vi "Write Subscribe Target.vi"(8 "error in (no error)":errorcluster, 10 "Subscribe Target":string, 11 "Subscriber in":refnum<class "Subscriber.lvclass">) -> (0 "error out":errorcluster, 3 "Subscriber out":refnum<class "Subscriber.lvclass">)   [LabVIEW 2024, in "Subscriber.lvclass"]
uses:
  Subscriber.lvclass
  Subscriber.lvclass/Subscriber.ctl
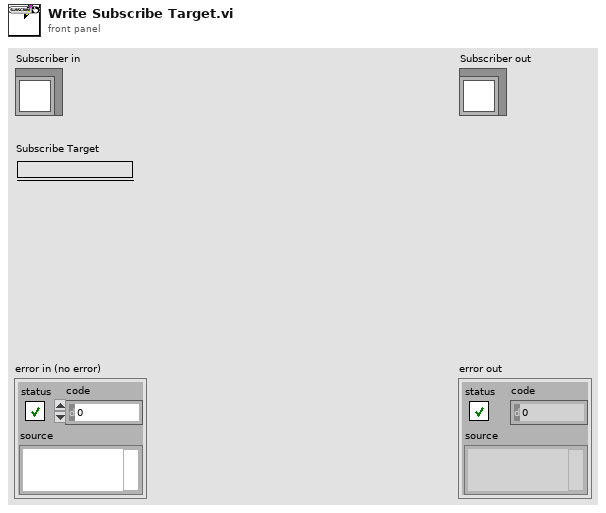
[diagram p1: front panel]
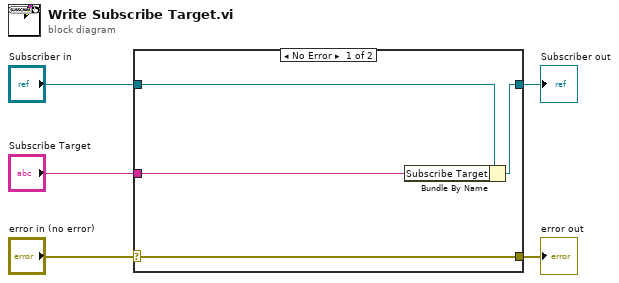
[diagram p0: block diagram]
diagram:
  n1 = case shown="No Error" "error in (no error)" {
    selector: "error in (no error)" -> [w9 w10]
    tunnel: [w9 w10] -> w4
    tunnel: [w7 w11] -> w2
    tunnel: "Subscriber in" -> [w8 w11]
    tunnel: "Subscribe Target" -> [w6 _]
    frame No Error {
      n2 = Bundle By Name(cluster=w8, "Subscribe Target"=w6) -> (w7:refnum<class "Subscriber.lvclass">)
    }
    frame Error {
    }
  }
  "error out" <- w4
  "Subscriber out" <- w2
